vi "SubPanel_DataCollection_Rev11_v2.vi"(0 "DCPowerInformationClusterArray_Input":T6(array[cluster]), 1 "VISAPowerInfoInputArray":T5(array[cluster]), 2 "Run Data SubPanel Input":T4, 3 "RF Block Parameters":T3, 4 "Oscilloscope Info Array":T2(array[cluster]) {"vertical coupling" items=["AC", "DC", "Ground"]}, 7 "error in":errorcluster) -> (20 "DCPowerInformationClusterArray_Output":T6(array[cluster]), 21 "VISAPowerInfoInputOutput":T5(array[cluster]), 22 "Run Data SubPanel Output":T4, 23 "RF Block Parameters Output":T3, 24 "Oscilloscope Info Array Output":T2(array[cluster]) {"vertical coupling" items=["AC", "DC", "Ground"]}, 25 "Reinitialize?":bool, 27 "error out":errorcluster)   [LabVIEW 2019]
uses:
  Controls/QueueDataControl.ctl
  Controls/DataBlockControl.ctl
  Controls/RFBlockControl.ctl
  <instrlib>/niScope/Controls/niScope vertical coupling.ctl
panel:
  in  "Time Array":timestamp[](array[timestamp])
  out "Full Run Information":string
  out "Ready For Next Run?":bool
  in  "Next Run":bool
  out "Latchup Output Data":dbl[][](array[numeric])
  out "Recording Data":bool
  out "Current 2":waveform(dbl)[](graph)
  out "Voltage 2":waveform(dbl)[](graph)
  out "Current":waveform(dbl)[](graph)
  out "Voltage":waveform(dbl)[](graph)
  in  "End Collecting":bool
  in  "Record Data Toggle":bool
  out "error of collection":errorcluster
  in  "force exit SubVI":bool
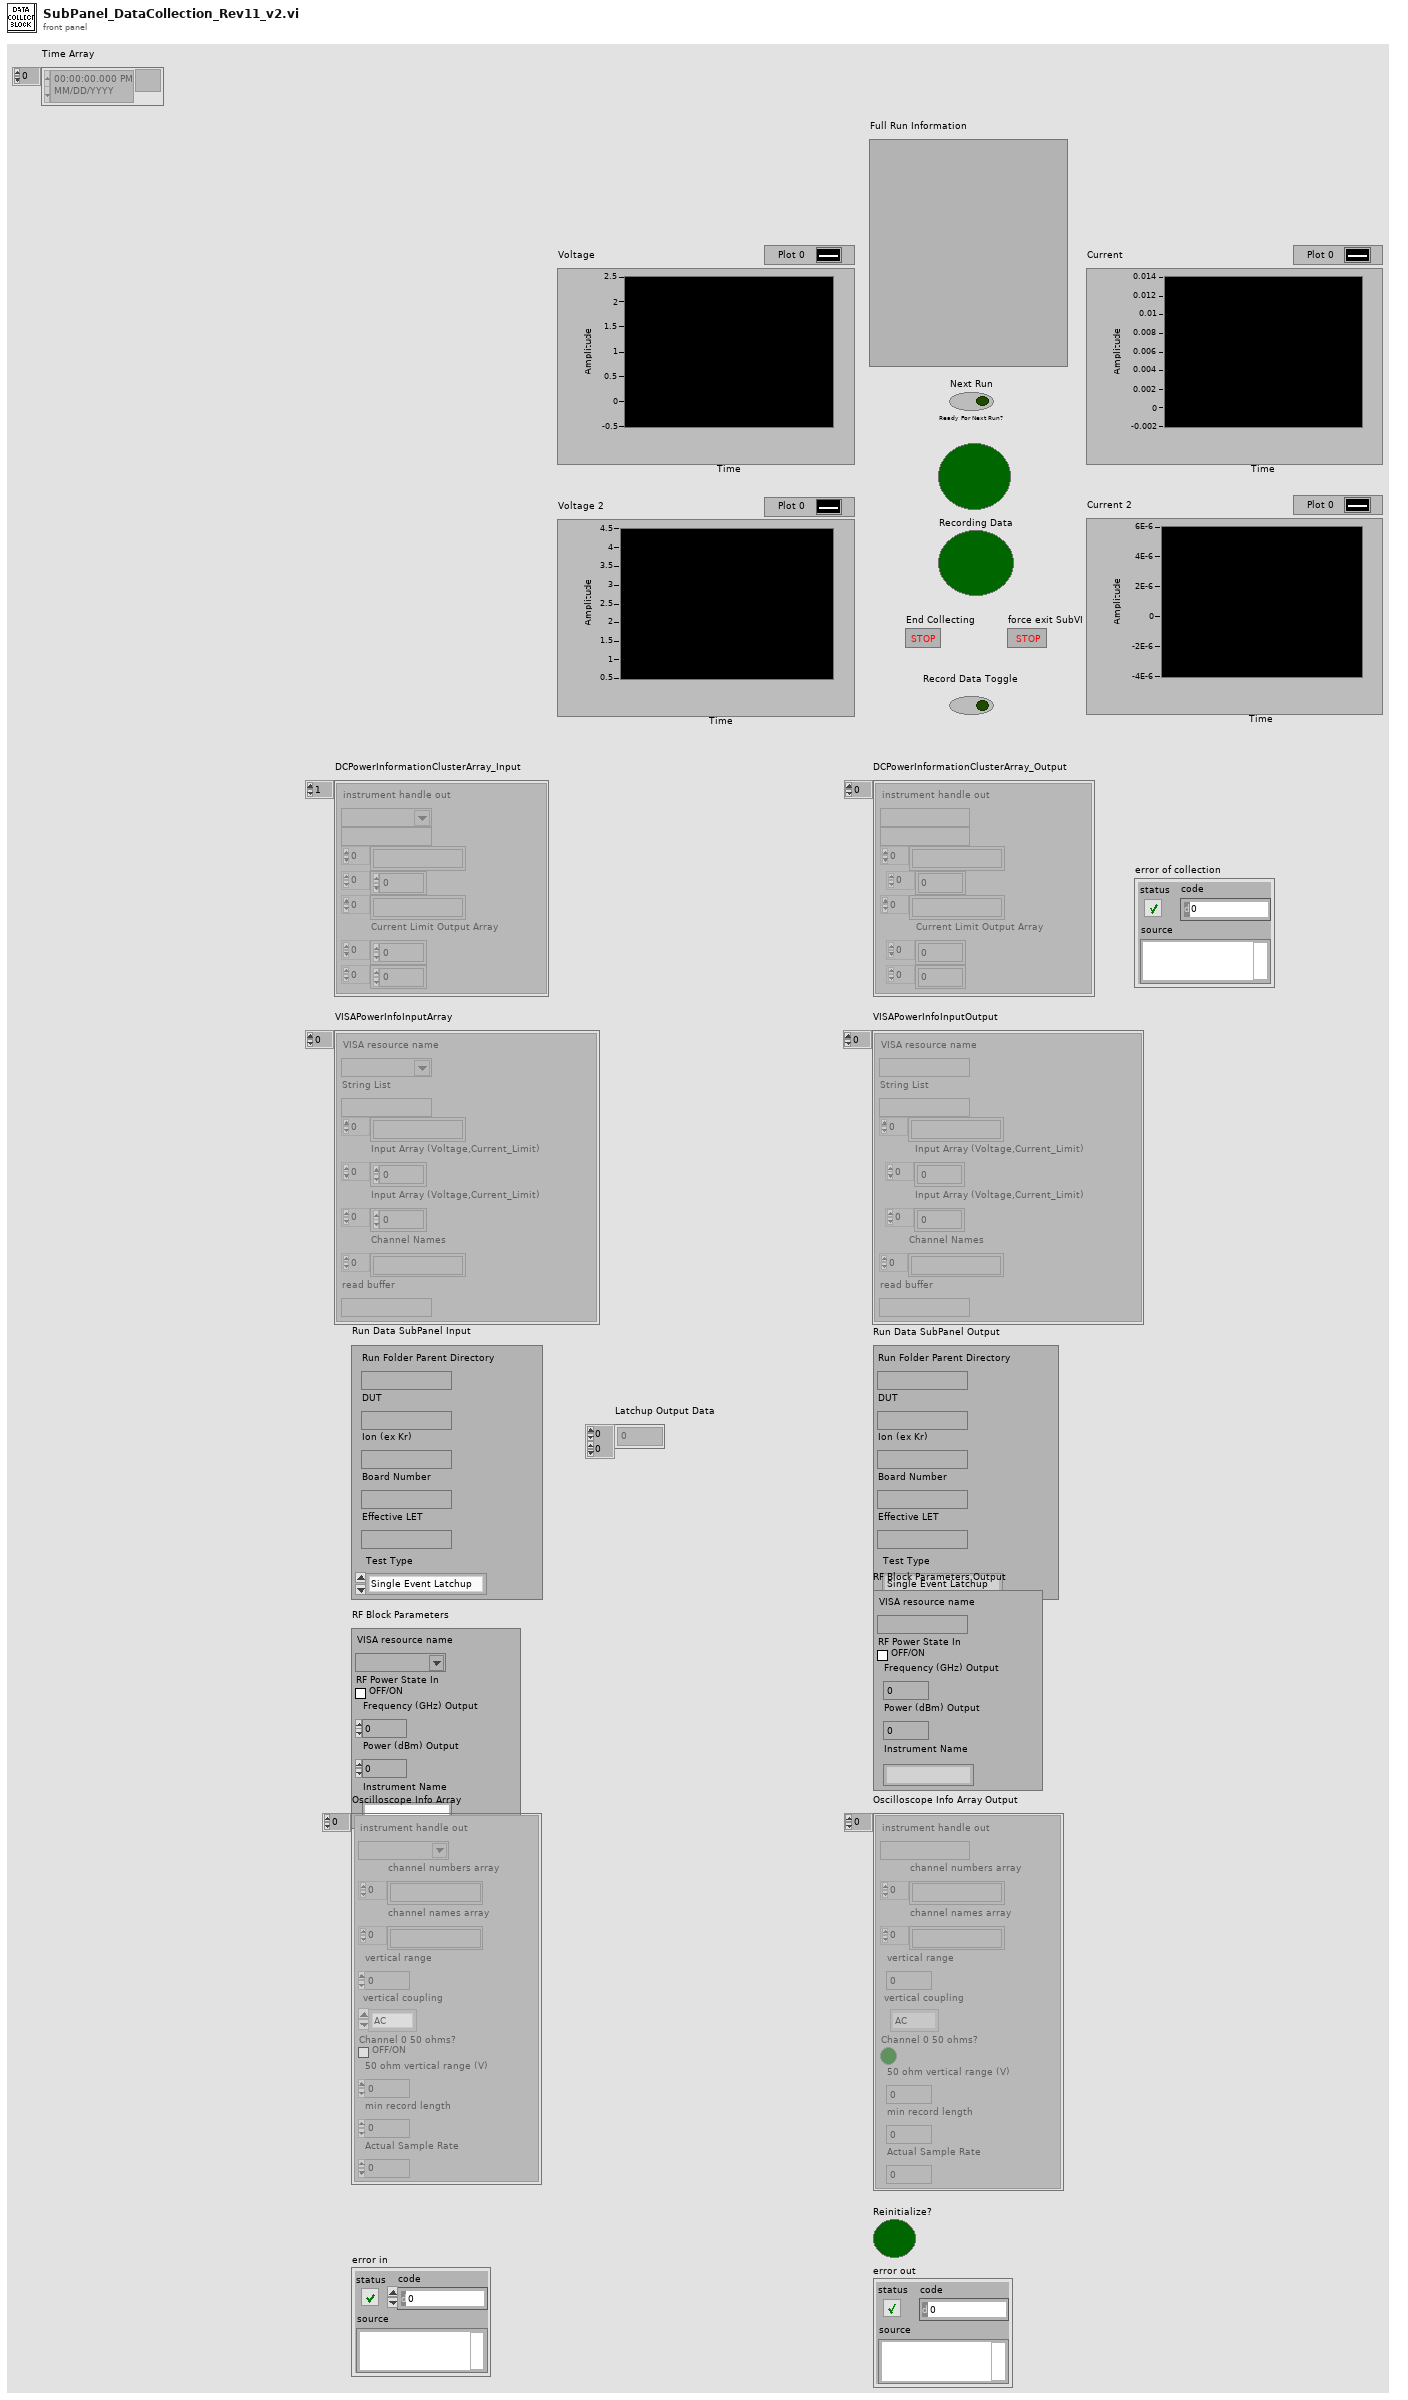
[diagram p1: front panel]
types:
  T1 = typedef "niScope vertical coupling.ctl" = i32
  T2 = cluster{"instrument handle out":refnum<k15>, "channel numbers array":string[], "channel names array":string[], "vertical range":dbl, "vertical coupling":T1, "Channel 0 50 ohms?":bool, "50 ohm vertical range (V)":dbl, "min record length":i32, "Actual Sample Rate":dbl}[]
  T3 = typedef "RFBlockControl.ctl" = cluster{"VISA resource name":refnum<visa-resource-name>, "RF Power State In":bool, "Frequency (GHz) Output":dbl, "Power (dBm) Output":dbl, "Instrument Name":string}
  T4 = typedef "DataBlockControl.ctl" = cluster{"Run Folder Parent Directory":path, "DUT":string, "Ion (ex Kr)":string, "Board Number":string, "Effective LET":string, "Test Type":enum16{"Single Event Latchup", "Single Event Transient", "Single Event Upset"}}
  T5 = cluster{"VISA resource name":refnum<visa-resource-name>, "String List":string, string[], "Input Array (Voltage,Current_Limit)":dbl[], "Input Array (Voltage,Current_Limit)":dbl[], "Channel Names":string[], "read buffer":string}[]
  T6 = cluster{"instrument handle out":refnum<k15>, string, string[], dbl[], string[], "Current Limit Output Array":dbl[], dbl[]}[]
  T7 = typedef "QueueDataControl.ctl" = cluster{"Rolling Timer":timestamp, "Initial Time":timestamp, "dt between samples":dbl[], "number of samples per fetch":i32[], "voltage measurements":dbl[][], "current measurements":dbl[][]}
  T8 = cluster{"IVI Refnum out":refnum<k15>, string, "voltage level channel 23":dbl, "Channel Name 23":string, "Current Limit":dbl, "Measure Record dt":dbl, string, "Current Threshold Reset Value Array":dbl}[]
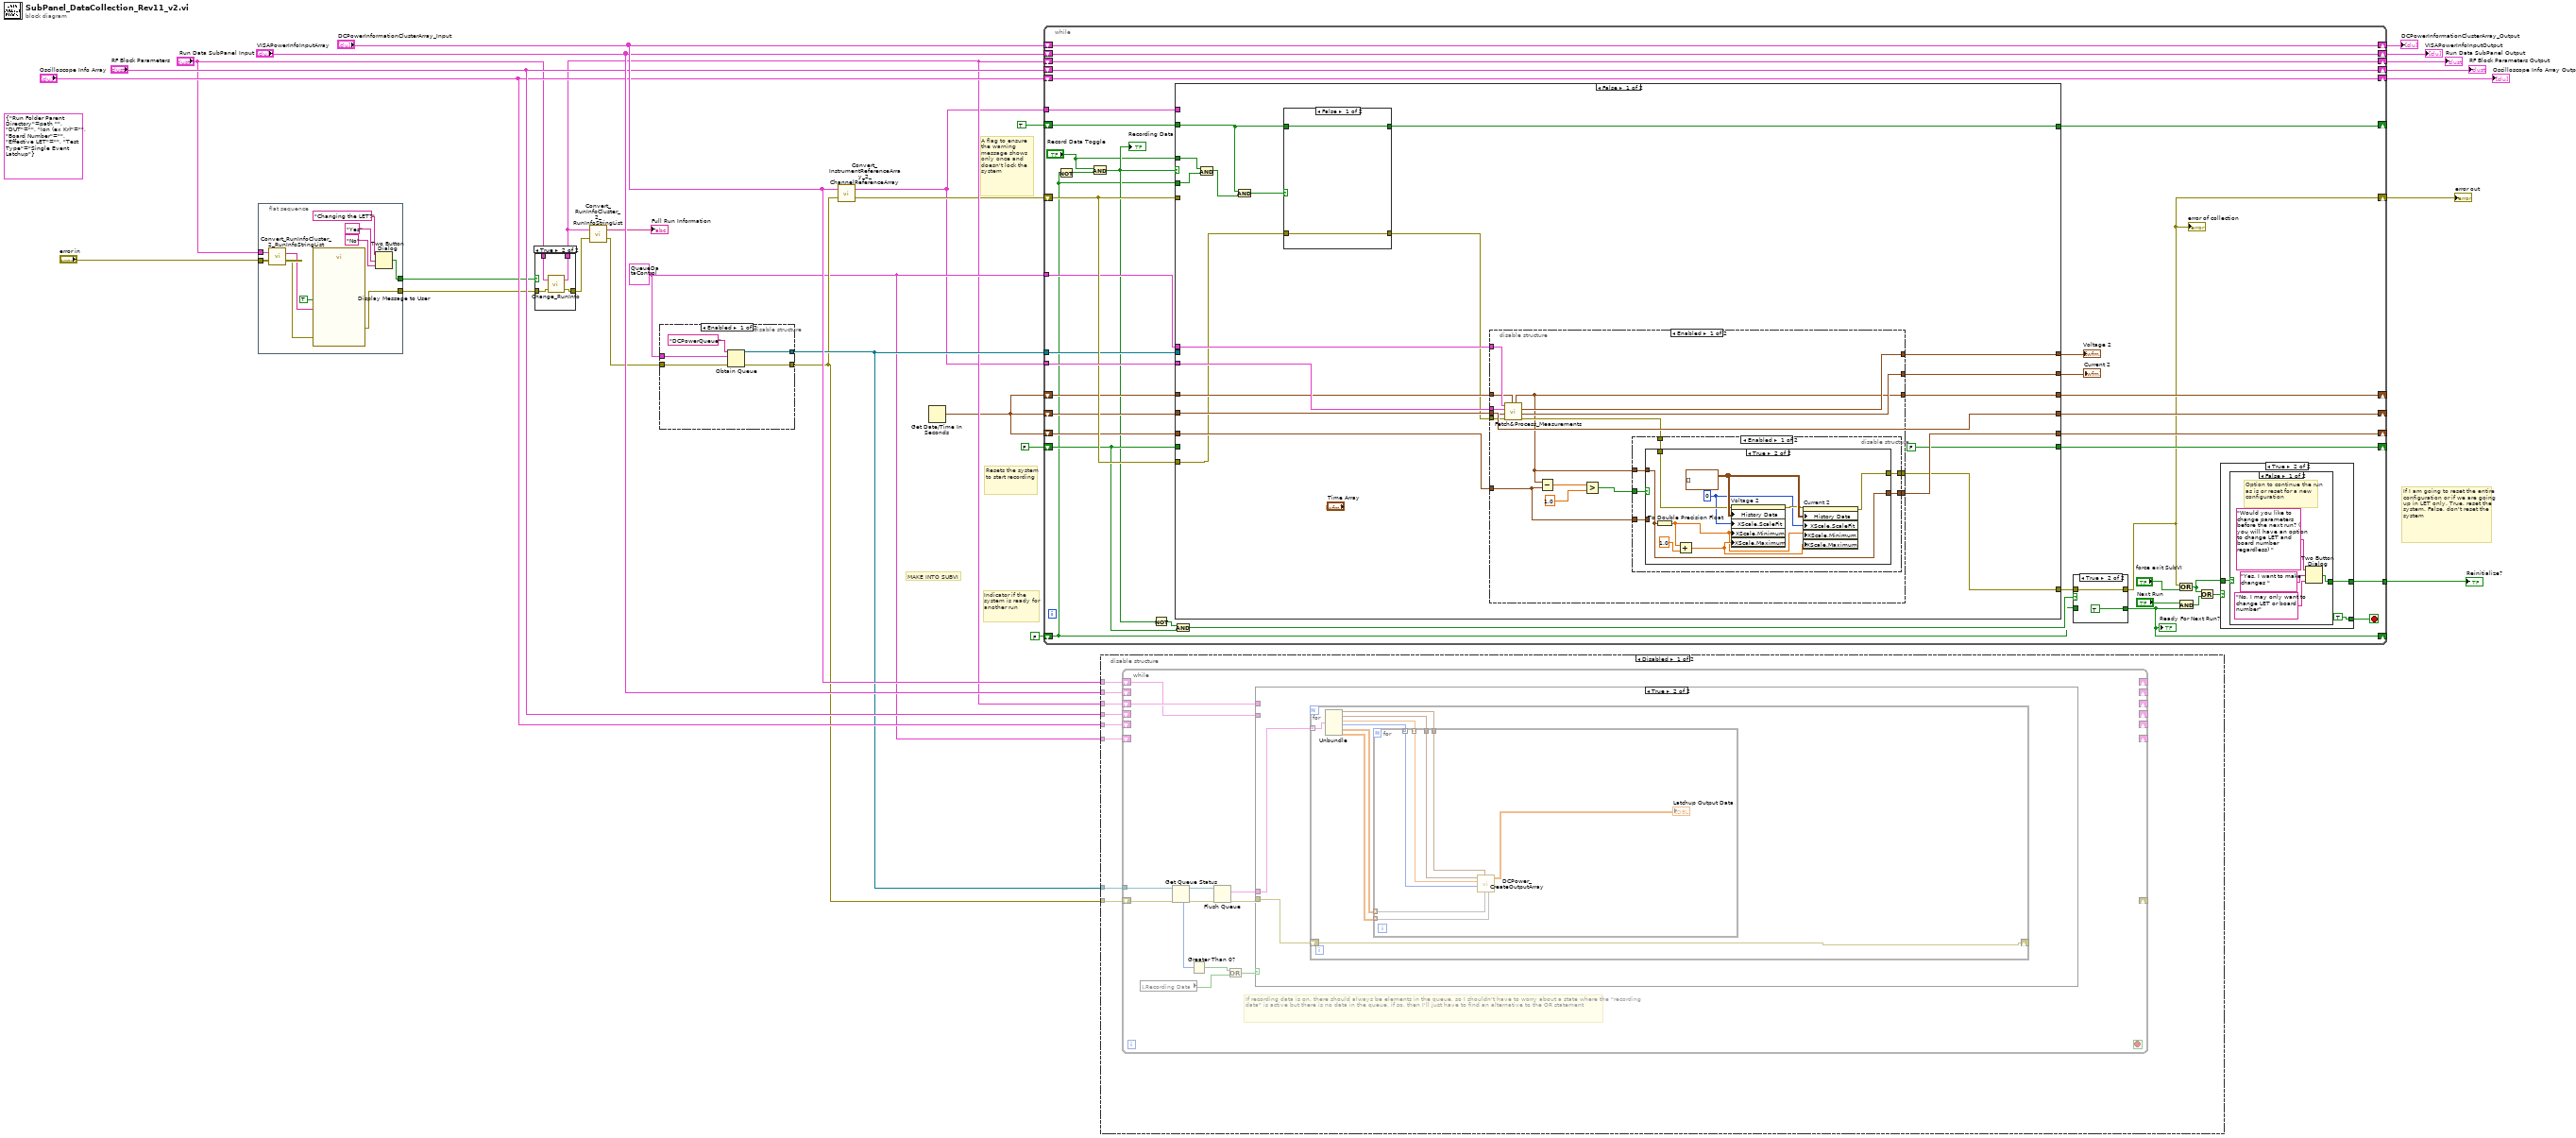
[diagram p0: block diagram]
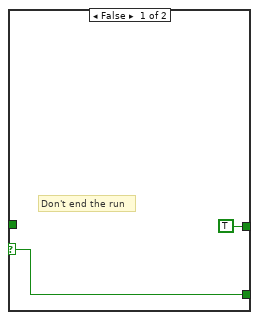
[diagram p6: hidden frame]
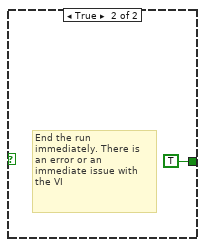
[diagram p7: hidden frame]
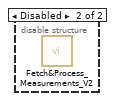
[diagram p11: hidden frame]
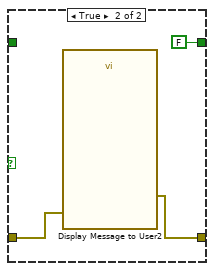
[diagram p12: hidden frame]
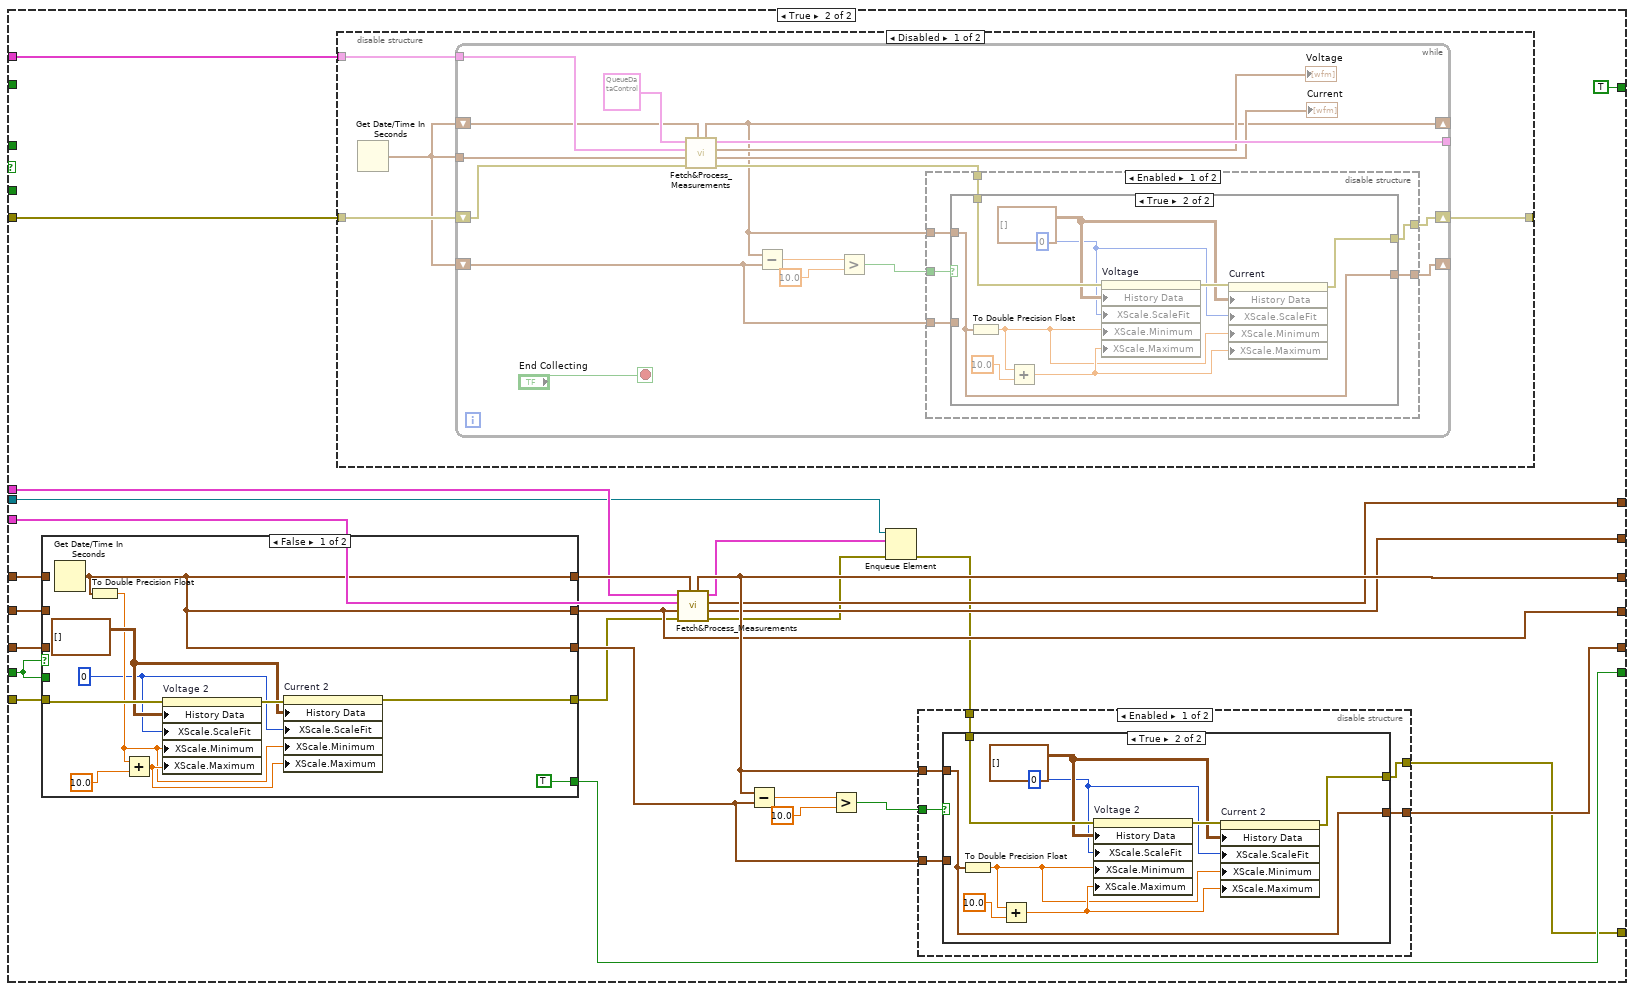
[diagram p13: hidden frame]
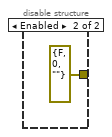
[diagram p16: hidden frame]
diagram:
  (unwired) T4 {"Run Folder Parent Directory"=path "", "DUT"="", "Ion (ex Kr)"="", "Board Number"="", "Effective LET"="", "Test Type"=enum."Single Event Latchup"} ("Run Data Configuration")
  w15 = T7 {"Rolling Timer"=timestamp(0 s since 1904-01-01), "Initial Time"=timestamp(0 s since 1904-01-01), "dt between samples"=[], "number of samples per fetch"=[], "voltage measurements"=[], "current measurements"=[]} ("Queue Data Parameters")
  # "Indicator if the system is ready for another run"
  # "Resets the system to start recording"
  # "A flag to ensure the warning message shows only once and doesn't lock the system"
  # "If I am going to reset the entire configuration or if we are going up in LET only. True, reset the system. False, don't reset the system"
  # "MAKE INTO SUBVI"
  n1 = flat-sequence {
    tunnel: [w34] -> w10
    tunnel: "error in" -> [w33]
    tunnel: [w38] -> w9
    tunnel: "Run Data SubPanel Input" -> [w31]
    frame #0 {
      n2 = call "Convert_RunInfoCluster_2_RunInfoStringList.vi"("error in"=w33, "Run Data SubPanel Input"=w31) -> ("error output"=w32:errorcluster, "Run Data Output"=w30:string)
      n3 = call "Display Message to User"("error in (no error)"=w32, "Enable"=TRUE, "Message"=w30) -> ("error out"=w34:errorcluster)  [unwired: 7 in, 1 out]
      n4 = Two Button Dialog(message="Changing the LET?", 1:"No" ("F button name (\"Cancel\")"), 2:"Yes" ("T button name (\"OK\")")) -> (T button?=w38:bool)
    }
  }
  n5 = case shown="True" w9 {
    tunnel: "Run Data SubPanel Input" -> [w40 w44]
    tunnel: [w40 w43] -> w8
    tunnel: [w39 w42] -> w6
    tunnel: w10 -> [w39 w41]
    frame False {
    }
    frame True {
      n6 = call "Change_RunInfo.vi"("error in (no error)"=w41, "Run Data SubPanel in"=w44) -> ("error out"=w42:errorcluster, "Run Data SubPanel out"=w43:T4)
    }
  }
  n7 = call "Convert_RunInfoCluster_2_RunInfoStringList.vi"("error in"=w6, "Run Data SubPanel Input"=w8) -> ("error output"=w5:errorcluster, "Run Data Output"=→"Full Run Information":string)
  n8 = disable-structure shown="Enabled" {
    disable-tunnel: w5 -> [w48 w50]
    disable-tunnel: [w47 w50] -> w16
    disable-tunnel: w15 -> [w46 _]
    disable-tunnel: [w45 _] -> w17
    frame Enabled {
      n9 = Obtain Queue(name (unnamed)="DCPowerQueue", element data type=w46, error in (no error)=w48) -> (queue out=w45:refnum<queue>, error out=w47:errorcluster)  [unwired: 2 in, 1 out]
    }
    frame Disabled {
    }
  }
  n10 = call "Convert_InstrumentReferenceArray_2_ChannelReferenceArray.vi"("error in (no error)"=w16, "DCPowerInformationClusterArray_Input"="DCPowerInformationClusterArray_Input") -> ("error out"=w2:errorcluster, "DCPowerInformationArrayOutput"=w1:T8)
  n11 = Get Date/Time In Seconds() -> (seconds since 1Jan1904=w3:timestamp)
  n12 = while {
    shift-right: [w84] -> w28
    shift-left: "DCPowerInformationClusterArray_Input" -> [w84]
    shift-right: [w88] -> w27
    shift-left: "VISAPowerInfoInputArray" -> [w88]
    shift-right: [w87] -> w26
    shift-left: w8 -> [w87]
    shift-right: [w86] -> w25
    shift-left: "RF Block Parameters" -> [w86]
    shift-right: [w85] -> w24
    shift-left: "Oscilloscope Info Array" -> [w85]
    shift-right: [w60] -> w23
    shift-left: w2 -> [w81]
    tunnel: w1 -> [w83]
    tunnel: w1 -> [w82]
    shift-right: [w77] -> _
    shift-left: w3 -> [w80]
    shift-right: [w76] -> _
    shift-left: w3 -> [w79]
    shift-right: [w75] -> _
    shift-left: w3 -> [w78]
    shift-right: [w72] -> _
    shift-left: FALSE -> [w68]
    tunnel: w15 -> [w71]
    tunnel: w17 -> [w70]
    shift-right: [w63] -> _
    shift-left: FALSE -> [w53]
    tunnel: [w57] -> w14
    shift-right: [w51] -> _
    shift-left: TRUE ("x .and. y?") -> [w52]
    stop <- w58 stop-if-true
    n13 = Not(x=w53) -> (.not. x?=w55:bool)
    n14 = And(x="Record Data Toggle", y=w55) -> (x .and. y?=w56:bool)
    "Recording Data" <- w56
    n15 = Not(x=w56) -> (.not. x?=w69:bool)
    n16 = And(x=w69, y=w68) -> (x .and. y?=w67:bool)
    n17 = case shown="False" w56 {
      tunnel: w81 -> [_ w187]
      tunnel: w83 -> [_ w186]
      tunnel: w82 -> [w121 w182]
      tunnel: w81 -> [w110 w167]
      tunnel: w80 -> [w119 w179]
      tunnel: w79 -> [w116 w178]
      tunnel: w78 -> [w117 w177]
      tunnel: [w113 w176] -> w77
      tunnel: [w118 w175] -> w76
      tunnel: [w117 w174] -> w75
      tunnel: [w114 w173] -> w74
      tunnel: [w115 w172] -> w73
      tunnel: w71 -> [w120 w171]
      tunnel: w68 -> [_ w169]
      tunnel: [FALSE w170] -> w72
      tunnel: w70 -> [_ w163]
      tunnel: [w111 w162] -> w66
      tunnel: "Record Data Toggle" -> [w107 _]
      tunnel: w53 -> [w108 _]
      tunnel: w52 -> [w103 _]
      tunnel: [w104 TRUE] -> w51
      frame False {
        n18 = And(x=w107, y=w108) -> (x .and. y?=w106:bool)
        n19 = And(x=w103, y=w106) -> (x .and. y?=w105:bool)
        n20 = case shown="False" w105 {
          tunnel: [w157 w159] -> w109
          tunnel: w110 -> [w157 w160]
          tunnel: [w156 FALSE] -> w104
          tunnel: w103 -> [w156 _]
          frame False {
          }
          frame True {
            n21 = call "Display Message to User2"("error in (no error)"=w160) -> ("error out"=w159:errorcluster)  [unwired: 9 in, 1 out]
          }
        }
        n22 = disable-structure shown="Enabled" {
          disable-tunnel: w121 -> [w132 _]
          disable-tunnel: w120 -> [w131 _]
          disable-tunnel: w119 -> [w130 _]
          disable-tunnel: [w129 _] -> w118
          disable-tunnel: w117 -> [w128 _]
          disable-tunnel: w116 -> [w127 _]
          disable-tunnel: [w126 _] -> w115
          disable-tunnel: [w125 _] -> w114
          disable-tunnel: [w124 _] -> w113
          disable-tunnel: [w123 _] -> w111
          disable-tunnel: w109 -> [w122 _]
          frame Enabled {
            n23 = call "Fetch&Process_Measurements.vi"("Rolling Timer Input"=w130, "error in (no error)"=w122, "Initial Time"=w128, "DCPowerInformation_byChannel"=w132, "Queue Data Parameters in"=w131) -> ("error out"=w133:errorcluster, "Current Measurement"=w125:waveform(dbl)[], "Voltage Measurement"=w126:waveform(dbl)[], "Rolling Timer Output"=w124:timestamp)  [unwired: 2 in, 1 out]
            n24 = Subtract(x=w124, y=w127) -> (x-y=w135:dbl)
            n25 = Greater?(x=w135, y=1.0) -> (0:w134:bool)
            n26 = disable-structure shown="Enabled" {
              disable-tunnel: w134 -> [w142 _]
              disable-tunnel: w133 -> [w141 w155]
              disable-tunnel: [w140 w155] -> w123
              disable-tunnel: [w139 w154] -> w129
              disable-tunnel: w124 -> [w138 w154]
              disable-tunnel: w127 -> [w137 _]
              frame Enabled {
                n27 = case shown="True" w142 {
                  tunnel: w141 -> [w144 w150]
                  tunnel: [w144 w148] -> w140
                  tunnel: [w143 w152] -> w139
                  tunnel: w138 -> [_ w152]
                  tunnel: w137 -> [w143 _]
                  frame False {
                  }
                  frame True {
                    w147 = u8 0 ("X Scale.Scale Fit")
                    w151 = waveform(dbl)[][] [] ("History Data")
                    n28 = To Double Precision Float(number=w152) -> (double precision float=w145:dbl)
                    n29 = Add(x=w145, y=1.0) -> (x+y=w146:dbl)
                    n30 = property on="Voltage 2" class="WFChart (strict)"(error in=w150, "History Data"=w151, "XScale.ScaleFit"=w147, "XScale.Minimum"=w145, "XScale.Maximum"=w146) -> (error out=w149:errorcluster)  [unwired: 1 in, 1 out]
                    n31 = property on="Current 2" class="WFChart (strict)"(error in=w149, "History Data"=w151, "XScale.ScaleFit"=w147, "XScale.Minimum"=w145, "XScale.Maximum"=w146) -> (error out=w148:errorcluster)  [unwired: 1 in, 1 out]
                  }
                }
              }
              frame Disabled {
              }
            }
          }
          frame Disabled {
            n32 = call "Fetch&Process_Measurements_V2.vi"() -> ()  [unwired: 7 in, 5 out]
          }
        }
      }
      frame True {
        n33 = case shown="False" w169 {
          tunnel: [w233 w242] -> w181
          tunnel: [w233 w241] -> w174
          tunnel: [w233 w243] -> w180
          tunnel: w179 -> [_ w243]
          tunnel: w178 -> [_ w242]
          tunnel: w177 -> [_ w241]
          tunnel: [TRUE w240] -> w170
          tunnel: w169 -> [_ w240]
          tunnel: [w236 w239] -> w168
          tunnel: w167 -> [w235 w239]
          frame False {
            w229 = u8 0 ("X Scale.Scale Fit")
            w234 = waveform(dbl)[][] [] ("History Data")
            n34 = Get Date/Time In Seconds() -> (seconds since 1Jan1904=w233:timestamp)
            n35 = To Double Precision Float(number=w233) -> (double precision float=w230:dbl)
            n36 = Add(x=w230, y=10.0) -> (x+y=w231:dbl)
            n37 = property on="Voltage 2" class="WFChart (strict)"(error in=w235, "History Data"=w234, "XScale.ScaleFit"=w229, "XScale.Minimum"=w230, "XScale.Maximum"=w231) -> (error out=w237:errorcluster)  [unwired: 1 in, 1 out]
            n38 = property on="Current 2" class="WFChart (strict)"(error in=w237, "History Data"=w234, "XScale.ScaleFit"=w229, "XScale.Minimum"=w230, "XScale.Maximum"=w231) -> (error out=w236:errorcluster)  [unwired: 1 in, 1 out]
          }
          frame True {
          }
        }
        n39 = disable-structure shown="Disabled" {
          disable-tunnel: w187 -> [w191 _]
          disable-tunnel: w186 -> [w190 _]
          disable-tunnel: [w189 errorcluster {"status"=FALSE, "code"=0, "source"=""} ("error out")] -> _
          frame Disabled {
            n40 = Get Date/Time In Seconds() -> (seconds since 1Jan1904=w188:timestamp)
            n41 = while {
              shift-right: [w195] -> w189
              shift-left: w191 -> [w206]
              tunnel: w190 -> [w207]
              tunnel: w188 -> [w203]
              shift-right: [w193] -> _
              shift-left: w188 -> [w204]
              tunnel: [w202] -> _
              shift-right: [w194] -> _
              shift-left: w188 -> [w192]
              stop <- "End Collecting" stop-if-true
              n42 = call "Fetch&Process_Measurements.vi"("Rolling Timer Input"=w204, "error in (no error)"=w206, "Initial Time"=w203, "DCPowerInformation_byChannel"=w207, "Queue Data Parameters in"=T7 {"Rolling Timer"=timestamp(0 s since 1904-01-01), "Initial Time"=timestamp(0 s since 1904-01-01), "dt between samples"=[], "number of samples per fetch"=[], "voltage measurements"=[], "current measurements"=[]} ("Queue Data Parameters")) -> ("error out"=w196:errorcluster, "Current Measurement"=→"Current":waveform(dbl)[], "Voltage Measurement"=→"Voltage":waveform(dbl)[], "Queue Data Parameters out"=w202:T7, "Rolling Timer Output"=w193:timestamp)  [unwired: 2 in]
              n43 = Subtract(x=w193, y=w192) -> (x-y=w198:dbl)
              n44 = Greater?(x=w198, y=10.0) -> (0:w197:bool)
              n45 = disable-structure shown="Enabled" {
                disable-tunnel: w197 -> [w214 _]
                disable-tunnel: w196 -> [w213 w227]
                disable-tunnel: [w212 w227] -> w195
                disable-tunnel: [w211 w226] -> w194
                disable-tunnel: w193 -> [w210 w226]
                disable-tunnel: w192 -> [w209 _]
                frame Enabled {
                  n46 = case shown="True" w214 {
                    tunnel: w213 -> [w216 w225]
                    tunnel: [w216 w223] -> w212
                    tunnel: [w215 w217] -> w211
                    tunnel: w210 -> [_ w217]
                    tunnel: w209 -> [w215 _]
                    frame False {
                    }
                    frame True {
                      w220 = u8 0 ("X Scale.Scale Fit")
                      w221 = waveform(dbl)[][] [] ("History Data")
                      n47 = To Double Precision Float(number=w217) -> (double precision float=w218:dbl)
                      n48 = Add(x=w218, y=10.0) -> (x+y=w219:dbl)
                      n49 = property on="Voltage" class="WFChart (strict)"(error in=w225, "History Data"=w221, "XScale.ScaleFit"=w220, "XScale.Minimum"=w218, "XScale.Maximum"=w219) -> (error out=w224:errorcluster)  [unwired: 1 in, 1 out]
                      n50 = property on="Current" class="WFChart (strict)"(error in=w224, "History Data"=w221, "XScale.ScaleFit"=w220, "XScale.Minimum"=w218, "XScale.Maximum"=w219) -> (error out=w223:errorcluster)  [unwired: 1 in, 1 out]
                    }
                  }
                }
                frame Disabled {
                }
              }
            }
          }
          frame Enabled {
          }
        }
        n51 = call "Fetch&Process_Measurements.vi"("Rolling Timer Input"=w180, "error in (no error)"=w168, "Initial Time"=w174, "DCPowerInformation_byChannel"=w182, "Queue Data Parameters in"=w171) -> ("error out"=w165:errorcluster, "Current Measurement"=w173:waveform(dbl)[], "Voltage Measurement"=w172:waveform(dbl)[], "Queue Data Parameters out"=w166:T7, "Rolling Timer Output"=w176:timestamp)  [unwired: 2 in]
        n52 = Subtract(x=w176, y=w181) -> (x-y=w184:dbl)
        n53 = Greater?(x=w184, y=10.0) -> (0:w183:bool)
        n54 = Enqueue Element(queue=w163, element=w166, error in (no error)=w165) -> (error out=w164:errorcluster)  [unwired: 1 in, 2 out]
        n55 = disable-structure shown="Enabled" {
          disable-tunnel: w183 -> [w249 _]
          disable-tunnel: w164 -> [w248 w262]
          disable-tunnel: [w247 w262] -> w162
          disable-tunnel: [w246 w261] -> w175
          disable-tunnel: w176 -> [w245 w261]
          disable-tunnel: w181 -> [w244 _]
          frame Enabled {
            n56 = case shown="True" w249 {
              tunnel: w248 -> [w251 w260]
              tunnel: [w251 w258] -> w247
              tunnel: [w250 w252] -> w246
              tunnel: w245 -> [_ w252]
              tunnel: w244 -> [w250 _]
              frame False {
              }
              frame True {
                w255 = u8 0 ("X Scale.Scale Fit")
                w256 = waveform(dbl)[][] [] ("History Data")
                n57 = To Double Precision Float(number=w252) -> (double precision float=w253:dbl)
                n58 = Add(x=w253, y=10.0) -> (x+y=w254:dbl)
                n59 = property on="Voltage 2" class="WFChart (strict)"(error in=w260, "History Data"=w256, "XScale.ScaleFit"=w255, "XScale.Minimum"=w253, "XScale.Maximum"=w254) -> (error out=w259:errorcluster)  [unwired: 1 in, 1 out]
                n60 = property on="Current 2" class="WFChart (strict)"(error in=w259, "History Data"=w256, "XScale.ScaleFit"=w255, "XScale.Minimum"=w253, "XScale.Maximum"=w254) -> (error out=w258:errorcluster)  [unwired: 1 in, 1 out]
              }
            }
          }
          frame Disabled {
          }
        }
      }
    }
    "Voltage 2" <- w73
    "Current 2" <- w74
    n61 = case shown="True" w67 {
      tunnel: w66 -> [w99 w101]
      tunnel: [w100 TRUE] -> w63
      tunnel: w53 -> [w100 _]
      tunnel: [w99 w101] -> w60
      frame False {
      }
      frame True {
      }
    }
    "error of collection" <- w60
    "Ready For Next Run?" <- w63
    n62 = Or(x=w60, y="force exit SubVI") -> (x .or. y?=w62:bool)
    n63 = And(x="Next Run", y=w63) -> (x .and. y?=w65:bool)
    n64 = Or(x=w62, y=w65) -> (x .or. y?=w64:bool)
    n65 = case shown="True" w64 {
      selector: w64 -> [w90 _]
      tunnel: w62 -> [_ w93]
      tunnel: [w90 TRUE] -> w58
      tunnel: [TRUE ("T button?") w91] -> w57
      frame False {
        # "Don't end the run"
      }
      frame True {
        n66 = case shown="False" w93 {
          tunnel: [w94 TRUE] -> w91
          frame False {
            # "Option to continue the run as is or reset for a new configuration"
            n67 = Two Button Dialog(message="Would you like to change parameters before the next run? ( you will have an option to change LET and board number regardless) ", 1:"No, I may only want to change LET or board number" ("F button name (\"Cancel\")"), 2:"Yes, I want to make changes " ("T button name (\"OK\")")) -> (T button?=w94:bool)
          }
          frame True {
            # "End the run immediately. There is an error or an immediate issue with the VI"
          }
        }
      }
    }
  }
  "DCPowerInformationClusterArray_Output" <- w28
  "VISAPowerInfoInputOutput" <- w27
  "Run Data SubPanel Output" <- w26
  "RF Block Parameters Output" <- w25
  "Oscilloscope Info Array Output" <- w24
  "error out" <- w23
  "Reinitialize?" <- w14
  n68 = disable-structure shown="Disabled" {
    disable-tunnel: "DCPowerInformationClusterArray_Input" -> [w270 _]
    disable-tunnel: "VISAPowerInfoInputArray" -> [w269 _]
    disable-tunnel: w8 -> [w268 _]
    disable-tunnel: "RF Block Parameters" -> [w267 _]
    disable-tunnel: "Oscilloscope Info Array" -> [w266 _]
    disable-tunnel: w17 -> [w265 _]
    disable-tunnel: w16 -> [w264 _]
    disable-tunnel: w15 -> [w263 _]
    frame Disabled {
      n69 = while {
        shift-right: _ -> [_]
        shift-left: w270 -> [w271]
        shift-right: _ -> [_]
        shift-left: w269 -> [_]
        shift-right: _ -> [_]
        shift-left: w268 -> [w272]
        shift-right: _ -> [_]
        shift-left: w267 -> [_]
        shift-right: _ -> [_]
        shift-left: w266 -> [_]
        tunnel: w265 -> [w274]
        shift-right: _ -> [_]
        shift-left: w264 -> [w273]
        shift-right: _ -> [_]
        shift-left: w263 -> [_]
        stop <- _ stop-if-true
        # "If recording data is on, there should always be elements in the queue, so I shouldn't have to worry about a state where the \"recording data\" is active but there is no data in the queue, if so, then I'll just have to find an alternative to the OR statement"
        n70 = local read "Recording Data"() -> (w279:bool)
        n71 = Get Queue Status(queue=w274, error in (no error)=w273) -> (queue out=w276:refnum<queue>, error out=w277:errorcluster, # elements in queue=w282:i32)  [unwired: 1 in, 5 out]
        n72 = Greater Than 0?(x=w282) -> (x > 0?=w280:bool)
        n73 = Flush Queue(queue=w276, error in (no error)=w277) -> (remaining elements=w275:T7[], error out=w278:errorcluster)  [unwired: 1 out]
        n74 = Or(x=w280, y=w279) -> (x .or. y?=w281:bool)
        n75 = case shown="True" w281 {
          tunnel: w275 -> [_ w284]
          tunnel: w278 -> [_ w283]
          tunnel: w272 -> [_ _]
          tunnel: w271 -> [_ _]
          frame False {
          }
          frame True {
            n76 = for {
              tunnel: w284 -> [w292] mode=indexing
              shift-right: [w291] -> _
              shift-left: w283 -> [w291]
              n77 = Unbundle(w292) -> ("Rolling Timer"=w285:timestamp, "Initial Time"=w286:timestamp, "dt between samples"=w290:dbl[], "number of samples per fetch"=w289:i32[], "voltage measurements"=w288:dbl[][], "current measurements"=w287:dbl[][])
              n78 = for {
                tunnel: w290 -> [w299] mode=indexing
                tunnel: w289 -> [w298] mode=indexing
                tunnel: w288 -> [w293] mode=indexing
                tunnel: w287 -> [w294] mode=indexing
                tunnel: w286 -> [w297]
                tunnel: w285 -> [w296]
                n79 = call "DCPower_CreateOutputArray.vi"("current measurements"=w294, "voltage measurements"=w293, "Rolling Timer"=w296, "actual count"=w298, "Measure Record dt"=w299, "Initial Time"=w297) -> ("Array"=→"Latchup Output Data":dbl[][])  [unwired: 5 in]
              }
            }
          }
        }
      }
    }
    frame Enabled {
    }
  }
